vi "configuration UI.vi"() -> ()   [LabVIEW 2013, in "TEC editor node.lvclass"]
uses:
  TEC editor node.lvclass
  <vilib>/NI/Configuration Framework/Node/NodeRef.ctl
  <vilib>/NI/Configuration Framework/Node/NISE_CEF_Node.lvclass
  <vilib>/NI/AMC/Message Queue.ctl
  <vilib>/NI/AMC/Message.ctl
  <vilib>/NI/Tools/Keyed Array/KeyedArray.ctl
  <vilib>/NI/Configuration Framework/Node/UserEventRef.ctl
  <vilib>/NI/Configuration Framework/Controls/EventCluster.ctl
  TEC editor node.lvclass/TEC editor node.ctl
  <vilib>/NI/Tag Bus/tag/Data Type.ctl
  <vilib>/NI/Tag Bus Module Framework/channel/channel classification.ctl
  <vilib>/NI/Tag Bus Module Framework/channel/TBM channel.lvclass/TBM channel.ctl
  <vilib>/NI/Configuration Framework/serializable configuration/NISE_CEF_serializable configuration.lvclass/NISE_CEF_serializable configuration.ctl
  <vilib>/NI/Configuration Framework/serializable configuration/NISE_CEF_serializable configuration.lvclass
  module/configuration/TEC configuration.lvclass
  <vilib>/NI/Tag Bus/tag/tag descriptor.lvclass/tag descriptor.ctl
  <vilib>/NI/Tag Bus Data Framework/Configuration Editor/Classes/Module editor node/Read display name.vi
  <vilib>/NI/Tag Bus Data Framework/Configuration Editor/Classes/Module editor node/module editor node.lvclass
  <vilib>/NI/Configuration Framework/NISE_CEF_TreeControl.lvlib
  <vilib>/NI/Tag Bus/tag/tag descriptor.lvclass
  <vilib>/NI/Module Execution Interface/Engine Configuration/engine configuration.lvclass
  <vilib>/NI/Tag Bus Module Framework/channel/TBM channel.lvclass
  <vilib>/NI/Tag Bus Data Framework/Configuration Editor/Classes/Engine Parent/Engine Parent Editor Node.lvclass
  <vilib>/NI/Tools/Keyed Array/Tools_KeyedArray.lvlib
  <vilib>/NI/AMC/AMC.lvlib
panel:
  in  "Tab Control":enum32{"Module Pairing", "Channel Mapping"}(tab)
  out "Guid":string
  in  "unpair":bool
  out "Paired with":string
  in  "pair":bool
  in  "Pairing Options":i32(listbox)
  in  "remove to":bool
  in  "add to":bool
  in  "toExtList":i32(listbox)
  in  "fromExternallist":i32(listbox)
  in  "avail tags":i32(listbox)=-1
  in  "user event":T1
  in  "main queue":T2
  in  "node ref":T3
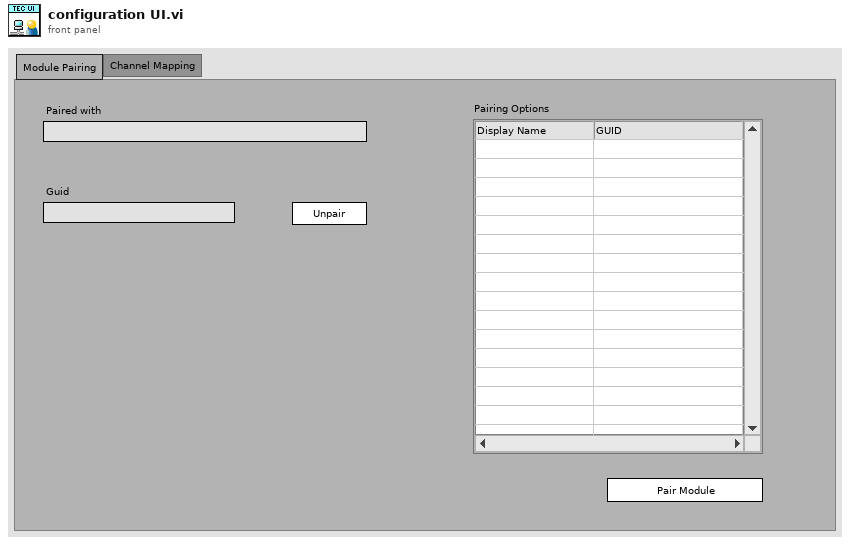
[diagram p1: front panel]
types:
  T1 = typedef "NISE_CEF_Node.lvclass/UserEventRef.ctl" = refnum<user-event>
  T2 = typedef "AMC.lvlib/Message Queue.ctl" = refnum<queue>
  T3 = typedef "NISE_CEF_Node.lvclass/NodeRef.ctl" = refnum<data-value>
  T4 = typedef "NISE_CEF_TreeControl.lvlib/EventCluster.ctl" = cluster{"command":string, "data":string}
  T5 = typedef "TBM channel.lvclass/channel classification.ctl" = enum16{"input data", "output data", "processing parameter", "processing result"}
  T6 = typedef "tag bus.lvlib/tag descriptor.lvclass/Data Type.ctl" = enum16{"Double", "Single", "I64", "I32", "I16", "I8", "U64", "U32", "U16", "U8", "Boolean", "String", "Array of Double", "Array of Single", "Array of I64", "Array of I32", "Array of I16", "Array of I8", "Array of U64", "Array of U32", "Array of U16", "Array of U8", "Array of Boolean", "Array of String"}
  T7 = typedef "TEC editor node.lvclass/pair information.ctl" = cluster{"paired guid":string}
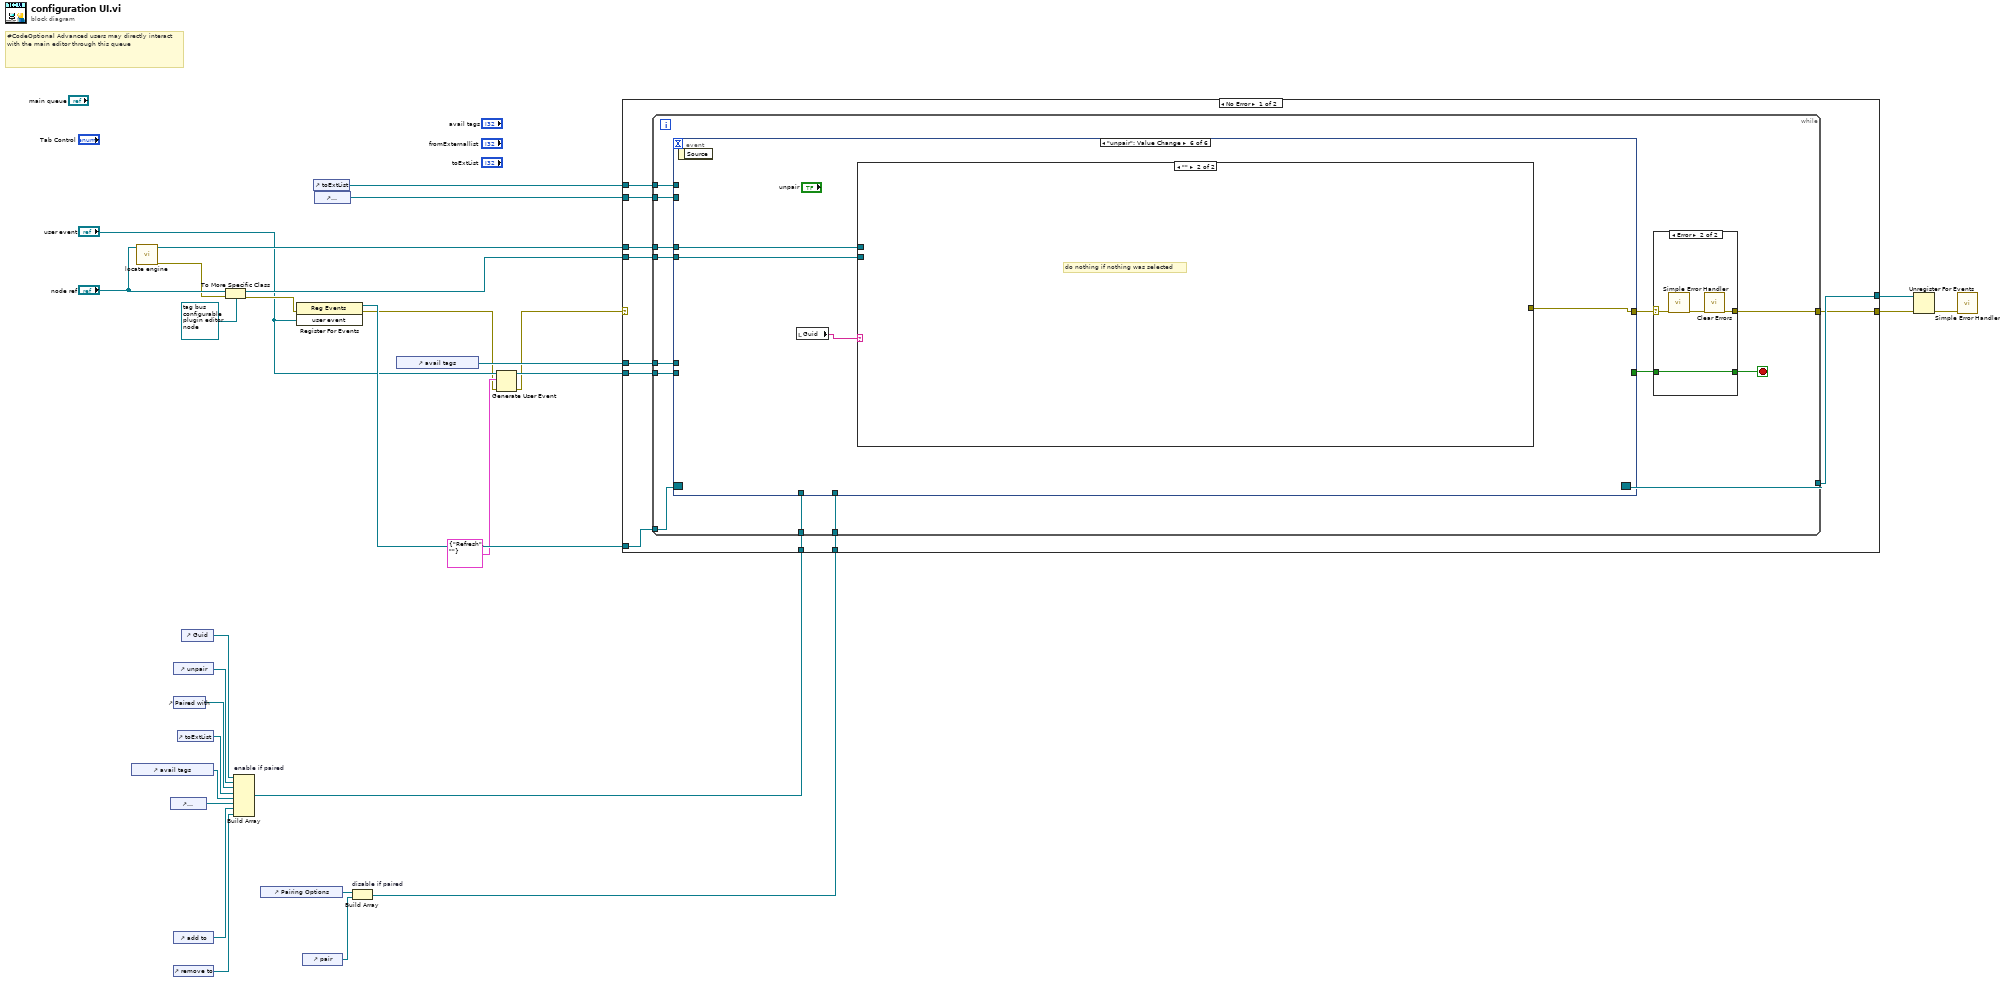
[diagram p0: block diagram]
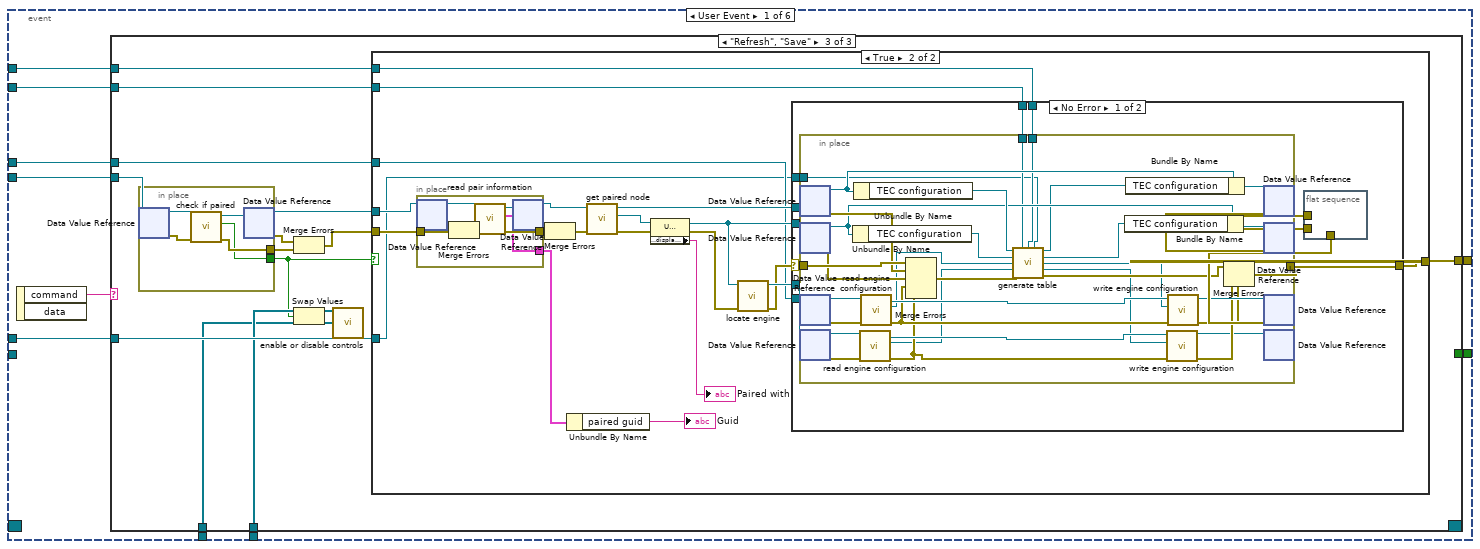
[diagram p3: hidden frame]
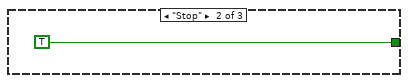
[diagram p5: hidden frame]
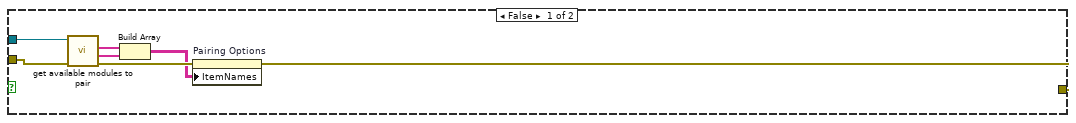
[diagram p6: hidden frame]
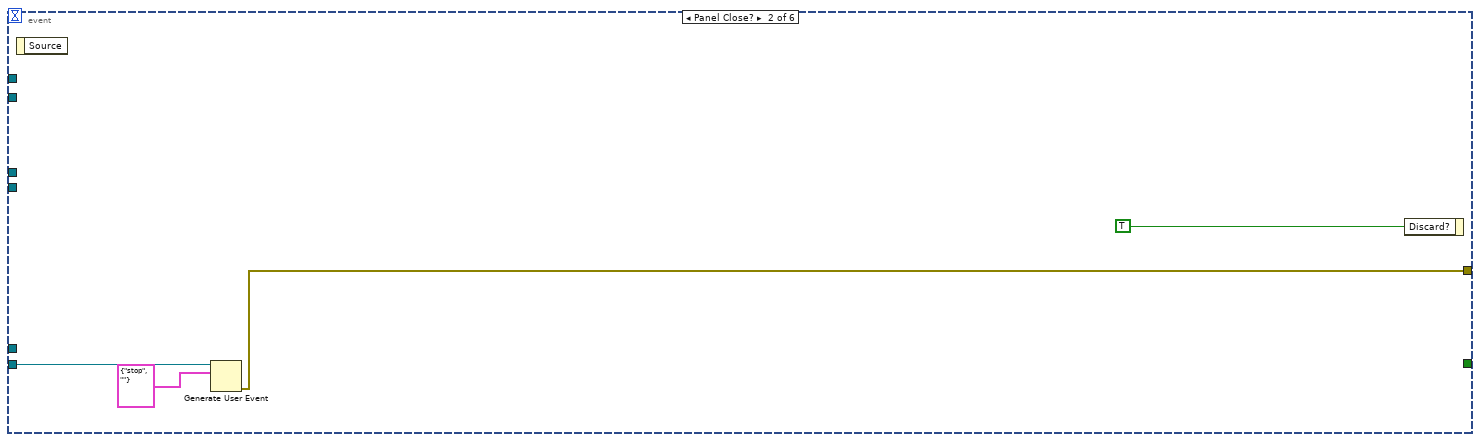
[diagram p8: hidden frame]
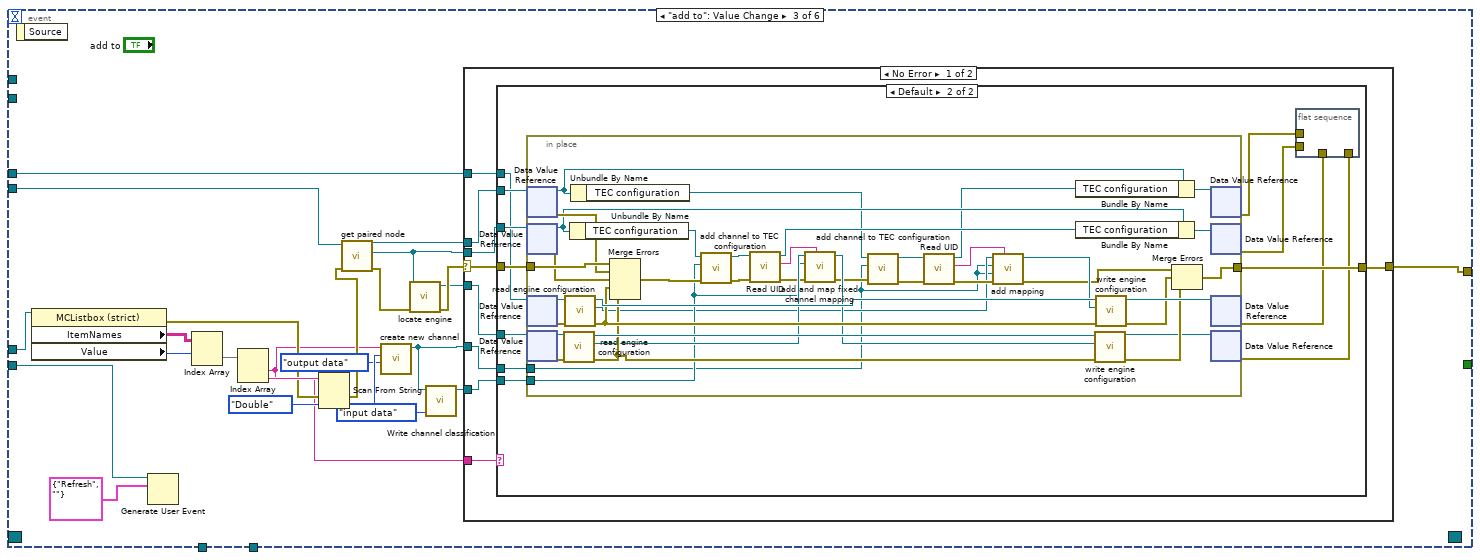
[diagram p9: hidden frame]
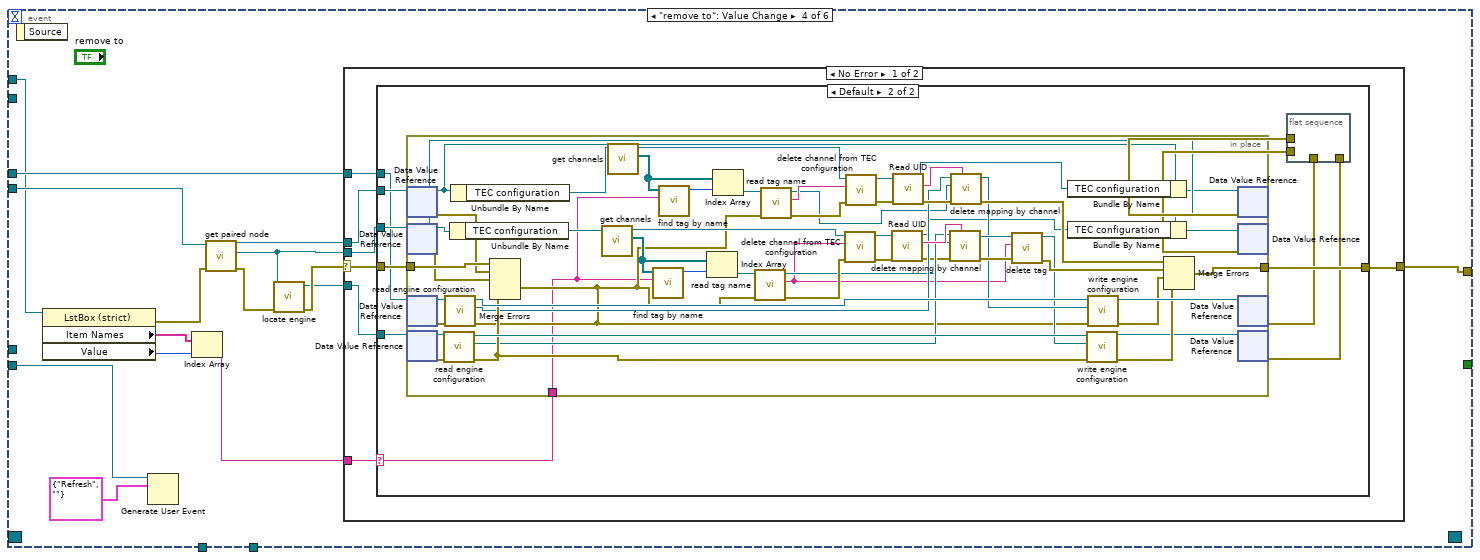
[diagram p12: hidden frame]
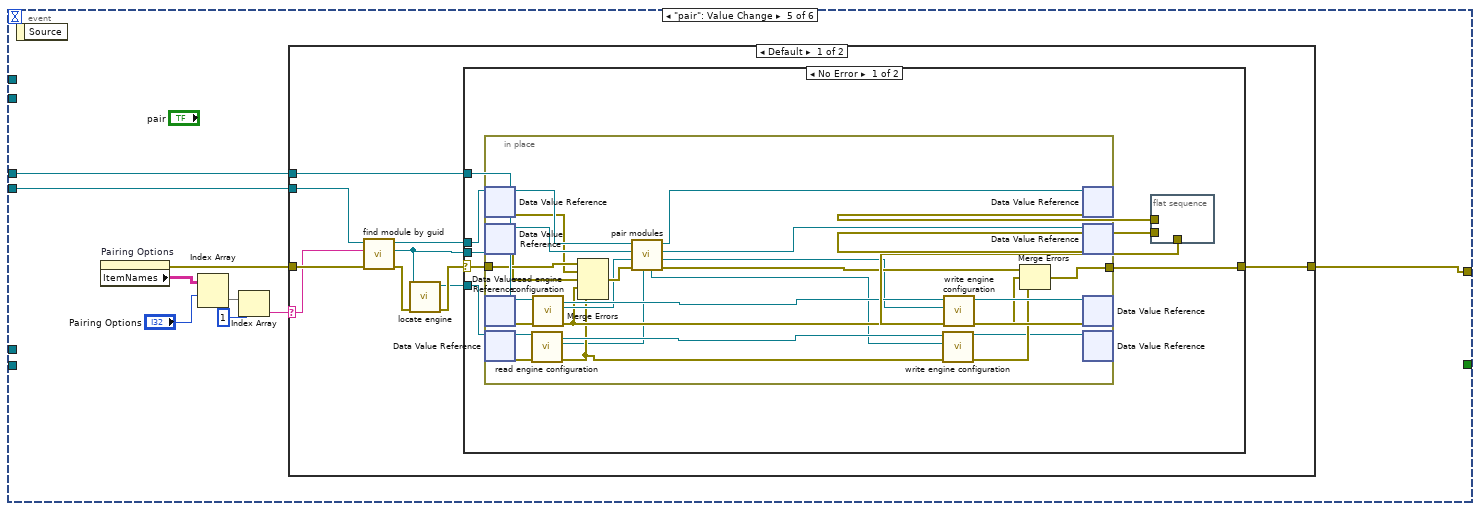
[diagram p15: hidden frame]
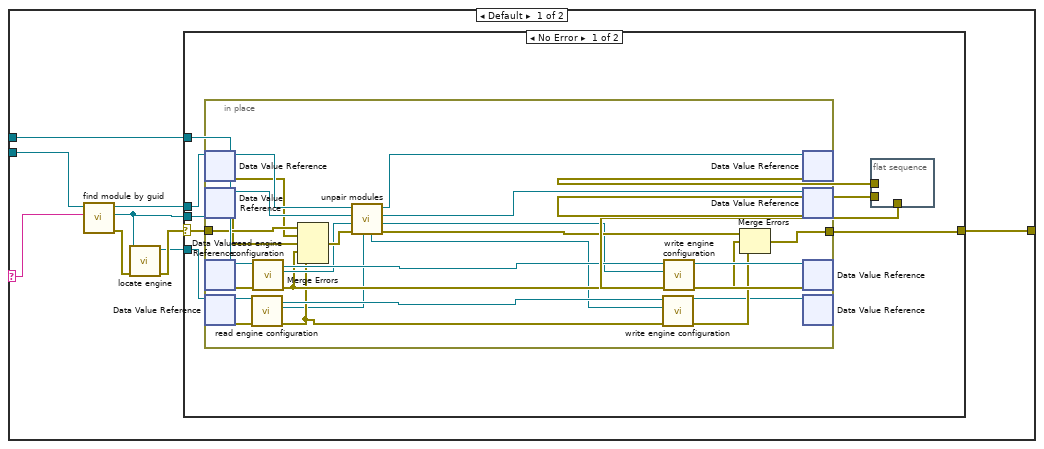
[diagram p18: hidden frame]
diagram:
  # "#CodeOptional Advanced users may directly interact with the main editor through this queue"
  n1 = control-ref of="avail tags"() -> (w10:refnum<vi>)
  n2 = call <vilib>:"locate engine.vi"("component"="node ref") -> ("error out"=w15:errorcluster, "engine"=w23:refnum<data-value>)  [unwired: 9 in]
  n3 = control-ref of="fromExternallist"() -> (w9:refnum<vi>)
  n4 = control-ref of="unpair"() -> (w13:refnum<vi>)
  n5 = control-ref of="Paired with"() -> (w14:refnum<vi>)
  n6 = control-ref of="add to"() -> (w7:refnum<vi>)
  n7 = control-ref of="remove to"() -> (w8:refnum<vi>)
  n8 = control-ref of="toExtList"() -> (w11:refnum<vi>)
  n9 = control-ref of="Guid"() -> (w12:refnum<vi>)
  n10 = To More Specific Class(target class=refnum<data-value> refnum ("data value reference"), reference="node ref", error in=w15) -> (specific class reference=w26:refnum<data-value>, error out=w25:errorcluster)
  n11 = Build Array "enable if paired"(w12, w13, w14, w11, w10, w9, w7, w8) -> (w5:refnum<vi>[])
  n12 = control-ref of="Pairing Options"() -> (w6:refnum<vi>)
  n13 = register-events(error in=w25, "user event") -> (reference out=w30:refnum<event-registration>, error out=w2:errorcluster)  [unwired: 1 in]
  n14 = control-ref of="pair"() -> (w3:refnum<vi>)
  n15 = control-ref of="toExtList"() -> (w21:refnum<vi>)
  n16 = control-ref of="fromExternallist"() -> (w1:refnum<vi>)
  n17 = Build Array "disable if paired"(w6, w3) -> (w4:refnum<vi>[])
  n18 = control-ref of="avail tags"() -> (w22:refnum<vi>)
  n19 = Generate User Event(user event="user event", event data cluster=T4 {"command"="Refresh", "data"=""} ("event data"), error in=w2) -> (user event out=w19:T1, error out=w17:errorcluster)  [unwired: 1 in]
  n20 = case shown="No Error" w17 {
    selector: w17 -> [_ w462]
    tunnel: w30 -> [w41 w461]
    tunnel: [w40 w461] -> w29
    tunnel: [w39 w462] -> w28
    tunnel: w26 -> [w38 _]
    tunnel: w23 -> [w37 _]
    tunnel: w22 -> [w36 _]
    tunnel: w21 -> [w35 _]
    tunnel: w19 -> [w34 _]
    tunnel: w5 -> [w33 _]
    tunnel: w4 -> [w32 _]
    tunnel: w1 -> [w31 _]
    frame No Error {
      n21 = while {
        tunnel: w41 -> [w55]
        tunnel: [w54] -> w40
        tunnel: w38 -> [w49]
        tunnel: w37 -> [w48]
        tunnel: w34 -> [w47]
        tunnel: w36 -> [w46]
        tunnel: w35 -> [w45]
        tunnel: [w50] -> w39
        tunnel: w33 -> [w44]
        tunnel: w32 -> [w43]
        tunnel: w31 -> [w42]
        stop <- w52 stop-if-true
        n22 = event shown="[5] \"unpair\": Value Change" {
          selector: w55 -> [_ _ _ _ _ _]
          dyn-events: [_ _ _ _ _ _] -> w54
          timeout: _ -> [_ _ _ _ _ _]
          tunnel: [w71 _ _ _ _ _] -> w51
          tunnel: [w69 w174 w201 w280 w357 w414] -> w53
          tunnel: w49 -> [w68 _ w197 w276 w359 w415]
          tunnel: w48 -> [w67 _ w200 w279 w356 w413]
          tunnel: w47 -> [_ w175 w192 w271 _ _]
          tunnel: w46 -> [w66 _ w186 _ _ _]
          tunnel: w45 -> [w65 _ _ w268 _ _]
          tunnel: w44 -> [w64 _ _ _ _ _]
          tunnel: w43 -> [w63 _ _ _ _ _]
          tunnel: w42 -> [w62 _ _ _ _ _]
          event User Event {
            n23 = event-data() -> ("command"=w70:string)  [unwired: 1 in, 1 out]
            n24 = case shown="\"Refresh\", \"Save\"" w70 {
              tunnel: [_ TRUE _] -> w71
              tunnel: [_ _ w84] -> w69
              tunnel: w68 -> [_ _ w83]
              tunnel: w67 -> [_ _ w85]
              tunnel: w66 -> [_ _ w87]
              tunnel: w65 -> [_ _ w86]
              tunnel: w64 -> [_ _ w77]
              tunnel: w63 -> [_ _ w78]
              tunnel: w62 -> [_ _ w73]
              frame Default {
              }
              frame "Stop" {
              }
              frame "Refresh", "Save" {
                n25 = in-place {
                  in-place-border: [w170] -> w80
                  in-place-border: [w169] -> w74
                  n26 = in-place-dvr #1(w83) -> (w173:refnum<class "TEC editor node.lvclass">, w171:errorcluster)
                  n27 = call "check if paired.vi"("error in"=w171, "UDP Broadcast Editor Node in"=w173) -> ("error out"=w170:errorcluster, "paired"=w169:bool, "UDP Broadcast Editor Node out"=w172:refnum<class "TEC editor node.lvclass">)  [unwired: 7 in]
                  n28 = in-place-dvr #1(w172) -> (w82:refnum<data-value>, w81:errorcluster)
                }
                n29 = Merge Errors(w81, w80) -> (w75:errorcluster)
                n30 = Swap Values(12:w78, 13:w74, 14:w77) -> (1:w79:refnum<vi>[], 3:w76:refnum<vi>[])
                n31 = call "enable or disable controls.vi"("disable set"=w76, "enable set"=w79) -> ()  [unwired: 10 in]
                n32 = case shown="True" w74 {
                  tunnel: w87 -> [_ w95]
                  tunnel: w86 -> [_ w96]
                  tunnel: w85 -> [_ w98]
                  tunnel: [w88 w102] -> w84
                  tunnel: w82 -> [w94 w105]
                  tunnel: w75 -> [w93 w106]
                  tunnel: w73 -> [_ w97]
                  frame False {
                    n33 = call "get available modules to pair.vi"("error in"=w93, "editor in"=w94) -> ("error out"=w90:errorcluster, "Display Name"=w92:string[], "IDs"=w91:string[])  [unwired: 6 in, 1 out]
                    n34 = Build Array(w91, w92) -> (w89:string[][])
                    n35 = property on="Pairing Options" class="MCListbox (strict)"(error in=w90, "ItemNames"=w89) -> (error out=w88:errorcluster)  [unwired: 1 in, 1 out]
                  }
                  frame True {
                    n36 = in-place {
                      in-place-border: w106 -> [w164]
                      in-place-border: [w168] -> w113
                      in-place-border: [w162] -> w108
                      n37 = in-place-dvr #2(w105) -> (w167:refnum<class "TEC editor node.lvclass">, w163:errorcluster)
                      n38 = Merge Errors(w164, w163) -> (w165:errorcluster)
                      n39 = call "read pair information.vi"("error in"=w165, "UDP Broadcast Editor Node in"=w167) -> ("error out"=w168:errorcluster, "pair info"=w162:T7, "UDP Broadcast Editor Node out"=w166:refnum<class "TEC editor node.lvclass">)  [unwired: 7 in]
                      n40 = in-place-dvr #2(w166) -> (w115:refnum<data-value>, w112:errorcluster)
                    }
                    n41 = Merge Errors(w113, w112) -> (w114:errorcluster)
                    n42 = Unbundle By Name(w108) -> ("paired guid"=→"Guid":string)
                    n43 = call "get paired node.vi"("error in"=w114, "editor in"=w115) -> ("error out"=w110:errorcluster, "paired node"=w111:refnum<data-value>, "editor out"=w100:refnum<data-value>)  [unwired: 7 in]
                    n44 = property class="UDP Broadcast Editor Node"(reference=w111, error in=w110) -> (reference out=w99:refnum<data-value>, error out=w101:errorcluster, "Data Access:display name"=→"Paired with":string)
                    n45 = call <vilib>:"locate engine.vi"("error in"=w101, "component"=w99) -> ("error out"=w103:errorcluster, "engine"=w104:refnum<data-value>)  [unwired: 8 in]
                    n46 = case shown="No Error" w103 {
                      selector: w103 -> [w127 w161]
                      tunnel: [w126 w161] -> w102
                      tunnel: w104 -> [w122 _]
                      tunnel: w100 -> [w121 _]
                      tunnel: w99 -> [w120 _]
                      tunnel: w98 -> [w119 _]
                      tunnel: w97 -> [w118 _]
                      tunnel: w96 -> [w117 _]
                      tunnel: w95 -> [w116 _]
                      frame No Error {
                        n47 = in-place {
                          in-place-border: w127 -> [w160]
                          in-place-border: [w153] -> w126
                          in-place-border: w118 -> [w130]
                          in-place-border: w117 -> [w129]
                          in-place-border: w116 -> [w128]
                          n48 = in-place-dvr #3(w121) -> (w136:refnum<class "TEC editor node.lvclass">, w159:errorcluster)
                          n49 = in-place-dvr #4(w120) -> (w133:refnum<class "TEC editor node.lvclass">, w158:errorcluster)
                          n50 = in-place-dvr #5(w119) -> (w157:refnum<class "Engine Parent Editor Node.lvclass">, w156:errorcluster)
                          n51 = in-place-dvr #6(w122) -> (w149:refnum<class "Engine Parent Editor Node.lvclass">, w148:errorcluster)
                          n52 = Unbundle By Name(w133) -> ("TEC configuration"=w137:refnum<class "TEC configuration.lvclass">)
                          n53 = Unbundle By Name(w136) -> ("TEC configuration"=w138:refnum<class "TEC configuration.lvclass">)
                          n54 = call <vilib>:"read engine configuration.vi"("error in"=w148, "Engine Parent Editor Node in"=w149) -> ("error out"=w147:errorcluster, "engine configuration"=w140:refnum<class "engine configuration.lvclass">, "Engine Parent Editor Node out"=w150:refnum<class "Engine Parent Editor Node.lvclass">)  [unwired: 7 in]
                          n55 = call <vilib>:"read engine configuration.vi"("error in"=w156, "Engine Parent Editor Node in"=w157) -> ("error out"=w151:errorcluster, "engine configuration"=w139:refnum<class "engine configuration.lvclass">, "Engine Parent Editor Node out"=w155:refnum<class "Engine Parent Editor Node.lvclass">)  [unwired: 7 in]
                          n56 = Merge Errors(w160, w159, w158, w151, w147) -> (w144:errorcluster)
                          n57 = call "generate table.vi"("TEC in"=w138, "from TEC"=w130, "to TEC"=w129, "avail tags"=w128, "Pair in"=w137, "engine configuration in"=w139, "paired engine in"=w140, "error in"=w144) -> ("TEC out"=w131:refnum<class "TEC configuration.lvclass">, "pair out"=w132:refnum<class "TEC configuration.lvclass">, "engine configuration out"=w141:refnum<class "engine configuration.lvclass">, "paired engine out"=w142:refnum<class "engine configuration.lvclass">, "error out"=w143:errorcluster)  [unwired: 3 in]
                          n58 = Bundle By Name(cluster=w133, "TEC configuration"=w132) -> (w134:refnum<class "TEC editor node.lvclass">)
                          n59 = Bundle By Name(cluster=w136, "TEC configuration"=w131) -> (w135:refnum<class "TEC editor node.lvclass">)
                          n60 = call <vilib>:"write engine configuration.vi"("error in"=w147, "engine configuration"=w142, "Engine Parent Editor Node in"=w150) -> ("error out"=w146:errorcluster, "Engine Parent Editor Node out"=w145:refnum<class "Engine Parent Editor Node.lvclass">)  [unwired: 7 in]
                          n61 = call <vilib>:"write engine configuration.vi"("error in"=w151, "engine configuration"=w141, "Engine Parent Editor Node in"=w155) -> ("error out"=w152:errorcluster, "Engine Parent Editor Node out"=w154:refnum<class "Engine Parent Editor Node.lvclass">)  [unwired: 7 in]
                          n62 = Merge Errors(w143, w152, w146) -> (w153:errorcluster)
                          n63 = in-place-dvr #3(w135) -> (w125:errorcluster)  [unwired: 1 out]
                          n64 = in-place-dvr #4(w134) -> (w124:errorcluster)  [unwired: 1 out]
                          n65 = in-place-dvr #5(w154) -> (w123:errorcluster)  [unwired: 1 out]
                          n66 = in-place-dvr #6(w145) -> ()  [unwired: 2 out]
                        }
                        n67 = flat-sequence {
                          tunnel: w125 -> [_]
                          tunnel: w124 -> [_]
                          tunnel: w123 -> [_]
                          frame #0 {
                          }
                        }
                      }
                      frame Error {
                      }
                    }
                  }
                }
              }
            }
          }
          event Panel Close? {
            n68 = event-data() -> ()  [unwired: 1 in, 1 out]
            n69 = Generate User Event(user event=w175, event data cluster=T4 {"command"="stop", "data"=""} ("event data")) -> (error out=w174:errorcluster)  [unwired: 2 in, 1 out]
            n70 = event-data("Discard?"=TRUE) -> ()  [unwired: 1 in, 1 out]
          }
          event "add to": Value Change {
            n71 = event-data() -> ()  [unwired: 1 in, 1 out]
            n72 = property class="MCListbox (strict)"(reference=w186) -> (error out=w184:errorcluster, "ItemNames"=w191:string[][], "Value"=w190:i32)  [unwired: 1 in, 1 out]
            n73 = Generate User Event(user event=w192, event data cluster=T4 {"command"="Refresh", "data"=""} ("event data")) -> ()  [unwired: 2 in, 2 out]
            n74 = Index Array(array=w191, index (row)=w190) -> (element=w187:string[])  [unwired: 1 in]
            n75 = Index Array(array=w187) -> (element #1=w178:string, element #2=w189:string)  [unwired: 2 in]
            n76 = Scan From String(input string=w189, error in=w184, default 1=Data_Type."Double" ("data type")) -> (error out=w185:errorcluster, output 1=w183:T6)  [unwired: 2 in, 2 out]
            n77 = call "get paired node.vi"("error in"=w185, "editor in"=w197) -> ("error out"=w194:errorcluster, "paired node"=w195:refnum<data-value>, "editor out"=w196:refnum<data-value>)  [unwired: 7 in]
            n78 = call <vilib>:"create new channel.vi"("channel classification"=channel_classification."output data", "data type"=w183, "channel name"=w178) -> ("channel"=w181:refnum<class "TBM channel.lvclass">)  [unwired: 8 in]
            n79 = call <vilib>:"locate engine.vi"("error in"=w194, "component"=w195) -> ("error out"=w199:errorcluster, "engine"=w198:refnum<data-value>)  [unwired: 8 in]
            n80 = call <vilib>:"Write channel classification.vi"("channel classification"=channel_classification."input data", "channel in"=w181) -> ("channel out"=w180:refnum<class "TBM channel.lvclass">)  [unwired: 8 in, 1 out]
            n81 = case shown="No Error" w199 {
              selector: w199 -> [w210 w265]
              tunnel: [w209 w265] -> w201
              tunnel: w196 -> [w208 _]
              tunnel: w195 -> [w207 _]
              tunnel: w200 -> [w206 _]
              tunnel: w198 -> [w205 _]
              tunnel: w181 -> [w202 _]
              tunnel: w180 -> [w203 _]
              tunnel: w178 -> [w204 _]
              frame No Error {
                n82 = case shown="Default" w204 {
                  tunnel: w210 -> [w211 w223]
                  tunnel: [w211 w222] -> w209
                  tunnel: w208 -> [_ w221]
                  tunnel: w207 -> [_ w220]
                  tunnel: w206 -> [_ w219]
                  tunnel: w205 -> [_ w216]
                  tunnel: w203 -> [_ w213]
                  tunnel: w202 -> [_ w212]
                  frame "" {
                  }
                  frame Default {
                    n83 = in-place {
                      in-place-border: w223 -> [w264]
                      in-place-border: [w257] -> w222
                      in-place-border: w213 -> [w242]
                      in-place-border: w212 -> [w226]
                      n84 = in-place-dvr #7(w221) -> (w247:refnum<class "TEC editor node.lvclass">, w263:errorcluster)
                      n85 = in-place-dvr #8(w220) -> (w246:refnum<class "TEC editor node.lvclass">, w262:errorcluster)
                      n86 = in-place-dvr #9(w219) -> (w261:refnum<class "Engine Parent Editor Node.lvclass">, w260:errorcluster)
                      n87 = in-place-dvr #10(w216) -> (w253:refnum<class "Engine Parent Editor Node.lvclass">, w252:errorcluster)
                      n88 = call <vilib>:"read engine configuration.vi"("error in"=w252, "Engine Parent Editor Node in"=w253) -> ("error out"=w251:errorcluster, "engine configuration"=w243:refnum<class "engine configuration.lvclass">, "Engine Parent Editor Node out"=w254:refnum<class "Engine Parent Editor Node.lvclass">)  [unwired: 7 in]
                      n89 = call <vilib>:"read engine configuration.vi"("error in"=w260, "Engine Parent Editor Node in"=w261) -> ("error out"=w255:errorcluster, "engine configuration"=w228:refnum<class "engine configuration.lvclass">, "Engine Parent Editor Node out"=w259:refnum<class "Engine Parent Editor Node.lvclass">)  [unwired: 7 in]
                      n90 = Unbundle By Name(w246) -> ("TEC configuration"=w244:refnum<class "TEC configuration.lvclass">)
                      n91 = Unbundle By Name(w247) -> ("TEC configuration"=w234:refnum<class "TEC configuration.lvclass">)
                      n92 = Merge Errors(w264, w263, w262, w255, w251) -> (w248:errorcluster)
                      n93 = call "add channel to TEC configuration.vi"("error in"=w248, "channel"=w242, "TEC configuration in"=w244) -> ("error out"=w241:errorcluster, "TEC configuration out"=w240:refnum<class "TEC configuration.lvclass">)  [unwired: 7 in]
                      n94 = call <vilib>:"Read UID.vi"("error in"=w241, "configuration in"=w240) -> ("error out"=w239:errorcluster, "instance id"=w238:string, "configuration out"=w237:refnum<class "TEC configuration.lvclass">)  [unwired: 7 in]
                      n95 = call <vilib>:"add and map fixed channel mapping.vi"("module instance"=w238, "error in"=w239, "fixed channel"=w242, "engine configuration in"=w243) -> ("error out"=w235:errorcluster, "engine configuration out"=w236:refnum<class "engine configuration.lvclass">)  [unwired: 6 in]
                      n96 = call "add channel to TEC configuration.vi"("error in"=w235, "channel"=w226, "TEC configuration in"=w234) -> ("error out"=w232:errorcluster, "TEC configuration out"=w233:refnum<class "TEC configuration.lvclass">)  [unwired: 7 in]
                      n97 = call <vilib>:"Read UID.vi"("error in"=w232, "configuration in"=w233) -> ("error out"=w231:errorcluster, "instance id"=w227:string, "configuration out"=w230:refnum<class "TEC configuration.lvclass">)  [unwired: 7 in]
                      n98 = call <vilib>:"add mapping.vi"("owner ID"=w227, "error in"=w231, "channel"=w226, "tag descriptor"=w226, "engine configuration"=w228) -> ("error out"=w225:errorcluster, "engine configuration out"=w229:refnum<class "engine configuration.lvclass">)  [unwired: 5 in]
                      n99 = Bundle By Name(cluster=w247, "TEC configuration"=w230) -> (w224:refnum<class "TEC editor node.lvclass">)
                      n100 = Bundle By Name(cluster=w246, "TEC configuration"=w237) -> (w245:refnum<class "TEC editor node.lvclass">)
                      n101 = call <vilib>:"write engine configuration.vi"("error in"=w251, "engine configuration"=w236, "Engine Parent Editor Node in"=w254) -> ("error out"=w250:errorcluster, "Engine Parent Editor Node out"=w249:refnum<class "Engine Parent Editor Node.lvclass">)  [unwired: 7 in]
                      n102 = call <vilib>:"write engine configuration.vi"("error in"=w255, "engine configuration"=w229, "Engine Parent Editor Node in"=w259) -> ("error out"=w256:errorcluster, "Engine Parent Editor Node out"=w258:refnum<class "Engine Parent Editor Node.lvclass">)  [unwired: 7 in]
                      n103 = Merge Errors(w225, w256, w250) -> (w257:errorcluster)
                      n104 = in-place-dvr #7(w224) -> (w218:errorcluster)  [unwired: 1 out]
                      n105 = in-place-dvr #8(w245) -> (w217:errorcluster)  [unwired: 1 out]
                      n106 = in-place-dvr #9(w258) -> (w215:errorcluster)  [unwired: 1 out]
                      n107 = in-place-dvr #10(w249) -> (w214:errorcluster)  [unwired: 1 out]
                    }
                    n108 = flat-sequence {
                      tunnel: w218 -> [_]
                      tunnel: w217 -> [_]
                      tunnel: w215 -> [_]
                      tunnel: w214 -> [_]
                      frame #0 {
                      }
                    }
                  }
                }
              }
              frame Error {
              }
            }
          }
          event "remove to": Value Change {
            n109 = event-data() -> ()  [unwired: 1 in, 1 out]
            n110 = property class="LstBox (strict)"(reference=w268) -> (error out=w267:errorcluster, "Item Names"=w270:string[], "Value"=w269:i32)  [unwired: 1 in, 1 out]
            n111 = Generate User Event(user event=w271, event data cluster=T4 {"command"="Refresh", "data"=""} ("event data")) -> ()  [unwired: 2 in, 2 out]
            n112 = Index Array(array=w270, index=w269) -> (element=w266:string)
            n113 = call "get paired node.vi"("error in"=w267, "editor in"=w276) -> ("error out"=w273:errorcluster, "paired node"=w274:refnum<data-value>, "editor out"=w275:refnum<data-value>)  [unwired: 7 in]
            n114 = call <vilib>:"locate engine.vi"("error in"=w273, "component"=w274) -> ("error out"=w278:errorcluster, "engine"=w277:refnum<data-value>)  [unwired: 8 in]
            n115 = case shown="No Error" w278 {
              selector: w278 -> [w287 w355]
              tunnel: [w286 w355] -> w280
              tunnel: w275 -> [w285 _]
              tunnel: w274 -> [w284 _]
              tunnel: w279 -> [w283 _]
              tunnel: w277 -> [w282 _]
              tunnel: w266 -> [w281 _]
              frame No Error {
                n116 = case shown="Default" w281 {
                  selector: w281 -> [_ w289]
                  tunnel: w287 -> [w288 w299]
                  tunnel: [w288 w298] -> w286
                  tunnel: w285 -> [_ w297]
                  tunnel: w284 -> [_ w296]
                  tunnel: w283 -> [_ w295]
                  tunnel: w282 -> [_ w292]
                  frame "" {
                  }
                  frame Default {
                    n117 = in-place {
                      in-place-border: w299 -> [w354]
                      in-place-border: [w347] -> w298
                      in-place-border: w289 -> [w301]
                      n118 = in-place-dvr #11(w297) -> (w339:refnum<class "TEC editor node.lvclass">, w353:errorcluster)
                      n119 = in-place-dvr #12(w296) -> (w338:refnum<class "TEC editor node.lvclass">, w352:errorcluster)
                      n120 = in-place-dvr #13(w295) -> (w351:refnum<class "Engine Parent Editor Node.lvclass">, w350:errorcluster)
                      n121 = in-place-dvr #14(w292) -> (w344:refnum<class "Engine Parent Editor Node.lvclass">, w343:errorcluster)
                      n122 = call <vilib>:"read engine configuration.vi"("error in"=w343, "Engine Parent Editor Node in"=w344) -> ("error out"=w342:errorcluster, "engine configuration"=w324:refnum<class "engine configuration.lvclass">, "Engine Parent Editor Node out"=w345:refnum<class "Engine Parent Editor Node.lvclass">)  [unwired: 7 in]
                      n123 = call <vilib>:"read engine configuration.vi"("error in"=w350, "Engine Parent Editor Node in"=w351) -> ("error out"=w307:errorcluster, "engine configuration"=w323:refnum<class "engine configuration.lvclass">, "Engine Parent Editor Node out"=w349:refnum<class "Engine Parent Editor Node.lvclass">)  [unwired: 7 in]
                      n124 = Unbundle By Name(w338) -> ("TEC configuration"=w314:refnum<class "TEC configuration.lvclass">)
                      n125 = Unbundle By Name(w339) -> ("TEC configuration"=w312:refnum<class "TEC configuration.lvclass">)
                      n126 = Merge Errors(w354, w353, w352, w307, w342) -> ()  [unwired: 1 out]
                      n127 = call-dynamic "get channels.vi"("TEC configuration in"=w314) -> ("channels"=w316:refnum<class "TBM channel.lvclass">[], "TEC configuration out"=w313:refnum<class "TEC configuration.lvclass">)  [unwired: 9 in]
                      n128 = call-dynamic "get channels.vi"("TEC configuration in"=w312) -> ("channels"=w319:refnum<class "TBM channel.lvclass">[], "TEC configuration out"=w311:refnum<class "TEC configuration.lvclass">)  [unwired: 9 in]
                      n129 = call <vilib>:"find tag by name.vi"("name"=w301, "tags in"=w316) -> ("index"=w315:i32)  [unwired: 9 in]
                      n130 = call <vilib>:"find tag by name.vi"("name"=w301, "tags in"=w319) -> ("index"=w318:i32)  [unwired: 9 in]
                      n131 = Index Array(array=w316, index=w315) -> (element=w317:refnum<class "TBM channel.lvclass">)
                      n132 = Index Array(array=w319, index=w318) -> (element=w320:refnum<class "TBM channel.lvclass">)
                      n133 = call <vilib>:"read tag name.vi"("error in"=w307, "system tag in"=w317) -> ("error out"=w308:errorcluster, "name"=w302:string, "system tag out"=w304:refnum<class "TBM channel.lvclass">)  [unwired: 7 in]
                      n134 = call <vilib>:"read tag name.vi"("error in"=w307, "system tag in"=w320) -> ("error out"=w309:errorcluster, "name"=w310:string, "system tag out"=w305:refnum<class "TBM channel.lvclass">)  [unwired: 7 in]
                      n135 = call "delete channel from TEC configuration.vi"("error in"=w308, "channel to delete"=w302, "TEC configuration in"=w313) -> ("error out"=w306:errorcluster, "TEC configuration out"=w333:refnum<class "TEC configuration.lvclass">)  [unwired: 7 in]
                      n136 = call "delete channel from TEC configuration.vi"("error in"=w309, "channel to delete"=w310, "TEC configuration in"=w311) -> ("error out"=w335:errorcluster, "TEC configuration out"=w336:refnum<class "TEC configuration.lvclass">)  [unwired: 7 in]
                      n137 = call <vilib>:"Read UID.vi"("error in"=w306, "configuration in"=w333) -> ("error out"=w303:errorcluster, "instance id"=w330:string, "configuration out"=w321:refnum<class "TEC configuration.lvclass">)  [unwired: 7 in]
                      n138 = call <vilib>:"Read UID.vi"("error in"=w335, "configuration in"=w336) -> ("error out"=w334:errorcluster, "instance id"=w329:string, "configuration out"=w322:refnum<class "TEC configuration.lvclass">)  [unwired: 7 in]
                      n139 = call <vilib>:"delete mapping by channel.vi"("owner ID"=w330, "error in"=w303, "channel"=w304, "engine configuration in"=w324) -> ("error out"=w331:errorcluster, "engine configuration out"=w332:refnum<class "engine configuration.lvclass">)  [unwired: 6 in]
                      n140 = call <vilib>:"delete mapping by channel.vi"("owner ID"=w329, "error in"=w334, "channel"=w305, "engine configuration in"=w323) -> ("error out"=w327:errorcluster, "engine configuration out"=w326:refnum<class "engine configuration.lvclass">)  [unwired: 6 in]
                      n141 = call <vilib>:"delete tag.vi"("error in"=w331, "tag name"=w302, "engine configuration in"=w332) -> ("error out"=w328:errorcluster, "engine configuration out"=w325:refnum<class "engine configuration.lvclass">)  [unwired: 7 in]
                      n142 = Bundle By Name(cluster=w339, "TEC configuration"=w322) -> (w300:refnum<class "TEC editor node.lvclass">)
                      n143 = Bundle By Name(cluster=w338, "TEC configuration"=w321) -> (w337:refnum<class "TEC editor node.lvclass">)
                      n144 = call <vilib>:"write engine configuration.vi"("error in"=w342, "engine configuration"=w325, "Engine Parent Editor Node in"=w345) -> ("error out"=w341:errorcluster, "Engine Parent Editor Node out"=w340:refnum<class "Engine Parent Editor Node.lvclass">)  [unwired: 7 in]
                      n145 = call <vilib>:"write engine configuration.vi"("error in"=w307, "engine configuration"=w326, "Engine Parent Editor Node in"=w349) -> ("error out"=w346:errorcluster, "Engine Parent Editor Node out"=w348:refnum<class "Engine Parent Editor Node.lvclass">)  [unwired: 7 in]
                      n146 = Merge Errors(w327, w328, w346, w341) -> (w347:errorcluster)
                      n147 = in-place-dvr #11(w300) -> (w294:errorcluster)  [unwired: 1 out]
                      n148 = in-place-dvr #12(w337) -> (w293:errorcluster)  [unwired: 1 out]
                      n149 = in-place-dvr #13(w348) -> (w291:errorcluster)  [unwired: 1 out]
                      n150 = in-place-dvr #14(w340) -> (w290:errorcluster)  [unwired: 1 out]
                    }
                    n151 = flat-sequence {
                      tunnel: w294 -> [_]
                      tunnel: w293 -> [_]
                      tunnel: w291 -> [_]
                      tunnel: w290 -> [_]
                      frame #0 {
                      }
                    }
                  }
                }
              }
              frame Error {
              }
            }
          }
          event "pair": Value Change {
            n152 = event-data() -> ()  [unwired: 1 in, 1 out]
            n153 = property on="Pairing Options" class="MCListbox (strict)"() -> (error out=w358:errorcluster, "ItemNames"=w364:string[][])  [unwired: 2 in, 1 out]
            n154 = Index Array(array=w364, index (row)="Pairing Options") -> (element=w362:string[])  [unwired: 1 in]
            n155 = Index Array(array=w362, index=1) -> (element=w360:string)
            n156 = case shown="Default" w360 {
              selector: w360 -> [w372 _]
              tunnel: w359 -> [w374 _]
              tunnel: w358 -> [w373 w411]
              tunnel: [w371 w411] -> w357
              tunnel: w356 -> [w369 _]
              frame Default {
                n157 = call "find module by guid.vi"("error in (no error)"=w373, "GUID"=w372, "ME in"=w374) -> ("error out"=w368:errorcluster, "UDP refs"=w366:refnum<data-value>, "ME out"=w370:refnum<data-value>)  [unwired: 6 in]
                n158 = call <vilib>:"locate engine.vi"("error in"=w368, "component"=w366) -> ("error out"=w367:errorcluster, "engine"=w365:refnum<data-value>)  [unwired: 8 in]
                n159 = case shown="No Error" w367 {
                  selector: w367 -> [w383 w410]
                  tunnel: [w382 w410] -> w371
                  tunnel: w370 -> [w381 _]
                  tunnel: w366 -> [w380 _]
                  tunnel: w369 -> [w379 _]
                  tunnel: w365 -> [w375 _]
                  frame No Error {
                    n160 = in-place {
                      in-place-border: w383 -> [w409]
                      in-place-border: [w394] -> w382
                      n161 = in-place-dvr #15(w381) -> (w406:refnum<class "TEC editor node.lvclass">, w404:errorcluster)
                      n162 = in-place-dvr #16(w380) -> (w407:refnum<class "TEC editor node.lvclass">, w403:errorcluster)
                      n163 = in-place-dvr #17(w379) -> (w400:refnum<class "Engine Parent Editor Node.lvclass">, w399:errorcluster)
                      n164 = in-place-dvr #18(w375) -> (w390:refnum<class "Engine Parent Editor Node.lvclass">, w389:errorcluster)
                      n165 = call <vilib>:"read engine configuration.vi"("error in"=w389, "Engine Parent Editor Node in"=w390) -> ("error out"=w388:errorcluster, "engine configuration"=w384:refnum<class "engine configuration.lvclass">, "Engine Parent Editor Node out"=w391:refnum<class "Engine Parent Editor Node.lvclass">)  [unwired: 7 in]
                      n166 = call <vilib>:"read engine configuration.vi"("error in"=w399, "Engine Parent Editor Node in"=w400) -> ("error out"=w392:errorcluster, "engine configuration"=w396:refnum<class "engine configuration.lvclass">, "Engine Parent Editor Node out"=w398:refnum<class "Engine Parent Editor Node.lvclass">)  [unwired: 7 in]
                      n167 = Merge Errors(w409, w404, w403, w392, w388) -> (w405:errorcluster)
                      n168 = call "pair modules.vi"("paired engine in"=w384, "error in"=w405, "engine configuration in"=w396, "module to pair with"=w407, "UDP Broadcast Editor Node in"=w406) -> ("error out"=w408:errorcluster, "engine configuration out"=w395:refnum<class "engine configuration.lvclass">, "module to pair with out"=w401:refnum<class "TEC editor node.lvclass">, "UDP Broadcast Editor Node out"=w402:refnum<class "TEC editor node.lvclass">, "paired engine out"=w385:refnum<class "engine configuration.lvclass">)  [unwired: 2 in]
                      n169 = call <vilib>:"write engine configuration.vi"("error in"=w388, "engine configuration"=w385, "Engine Parent Editor Node in"=w391) -> ("error out"=w387:errorcluster, "Engine Parent Editor Node out"=w386:refnum<class "Engine Parent Editor Node.lvclass">)  [unwired: 7 in]
                      n170 = call <vilib>:"write engine configuration.vi"("error in"=w392, "engine configuration"=w395, "Engine Parent Editor Node in"=w398) -> ("error out"=w393:errorcluster, "Engine Parent Editor Node out"=w397:refnum<class "Engine Parent Editor Node.lvclass">)  [unwired: 7 in]
                      n171 = Merge Errors(w408, w393, w387) -> (w394:errorcluster)
                      n172 = in-place-dvr #15(w402) -> (w378:errorcluster)  [unwired: 1 out]
                      n173 = in-place-dvr #16(w401) -> (w377:errorcluster)  [unwired: 1 out]
                      n174 = in-place-dvr #17(w397) -> (w376:errorcluster)  [unwired: 1 out]
                      n175 = in-place-dvr #18(w386) -> ()  [unwired: 2 out]
                    }
                    n176 = flat-sequence {
                      tunnel: w378 -> [_]
                      tunnel: w377 -> [_]
                      tunnel: w376 -> [_]
                      frame #0 {
                      }
                    }
                  }
                  frame Error {
                  }
                }
              }
              frame "" {
                # "do nothing if nothing was selected"
              }
            }
          }
          event "unpair": Value Change {
            n177 = event-data() -> ()  [unwired: 1 in, 1 out]
            n178 = local read "Guid"() -> (w412:string)
            n179 = case shown="\"\"" w412 {
              selector: w412 -> [w423 _]
              tunnel: w415 -> [w424 _]
              tunnel: [w422 _] -> w414
              tunnel: w413 -> [w420 _]
              frame Default {
                n180 = call "find module by guid.vi"("GUID"=w423, "ME in"=w424) -> ("error out"=w419:errorcluster, "UDP refs"=w417:refnum<data-value>, "ME out"=w421:refnum<data-value>)  [unwired: 7 in]
                n181 = call <vilib>:"locate engine.vi"("error in"=w419, "component"=w417) -> ("error out"=w418:errorcluster, "engine"=w416:refnum<data-value>)  [unwired: 8 in]
                n182 = case shown="No Error" w418 {
                  selector: w418 -> [w433 w460]
                  tunnel: [w432 w460] -> w422
                  tunnel: w421 -> [w431 _]
                  tunnel: w417 -> [w430 _]
                  tunnel: w420 -> [w429 _]
                  tunnel: w416 -> [w425 _]
                  frame No Error {
                    n183 = in-place {
                      in-place-border: w433 -> [w459]
                      in-place-border: [w444] -> w432
                      n184 = in-place-dvr #19(w431) -> (w456:refnum<class "TEC editor node.lvclass">, w454:errorcluster)
                      n185 = in-place-dvr #20(w430) -> (w457:refnum<class "TEC editor node.lvclass">, w453:errorcluster)
                      n186 = in-place-dvr #21(w429) -> (w450:refnum<class "Engine Parent Editor Node.lvclass">, w449:errorcluster)
                      n187 = in-place-dvr #22(w425) -> (w440:refnum<class "Engine Parent Editor Node.lvclass">, w439:errorcluster)
                      n188 = call <vilib>:"read engine configuration.vi"("error in"=w439, "Engine Parent Editor Node in"=w440) -> ("error out"=w438:errorcluster, "engine configuration"=w434:refnum<class "engine configuration.lvclass">, "Engine Parent Editor Node out"=w441:refnum<class "Engine Parent Editor Node.lvclass">)  [unwired: 7 in]
                      n189 = call <vilib>:"read engine configuration.vi"("error in"=w449, "Engine Parent Editor Node in"=w450) -> ("error out"=w442:errorcluster, "engine configuration"=w446:refnum<class "engine configuration.lvclass">, "Engine Parent Editor Node out"=w448:refnum<class "Engine Parent Editor Node.lvclass">)  [unwired: 7 in]
                      n190 = Merge Errors(w459, w454, w453, w442, w438) -> (w455:errorcluster)
                      n191 = call "unpair modules.vi"("paired engine in"=w434, "error in"=w455, "engine configuration in"=w446, "module to unpair"=w457, "UDP Broadcast Editor Node in"=w456) -> ("error out"=w458:errorcluster, "engine configuration out"=w445:refnum<class "engine configuration.lvclass">, "unpaired module"=w451:refnum<class "TEC editor node.lvclass">, "UDP Broadcast Editor Node out"=w452:refnum<class "TEC editor node.lvclass">, "paired engine out"=w435:refnum<class "engine configuration.lvclass">)  [unwired: 2 in]
                      n192 = call <vilib>:"write engine configuration.vi"("error in"=w438, "engine configuration"=w435, "Engine Parent Editor Node in"=w441) -> ("error out"=w437:errorcluster, "Engine Parent Editor Node out"=w436:refnum<class "Engine Parent Editor Node.lvclass">)  [unwired: 7 in]
                      n193 = call <vilib>:"write engine configuration.vi"("error in"=w442, "engine configuration"=w445, "Engine Parent Editor Node in"=w448) -> ("error out"=w443:errorcluster, "Engine Parent Editor Node out"=w447:refnum<class "Engine Parent Editor Node.lvclass">)  [unwired: 7 in]
                      n194 = Merge Errors(w458, w443, w437) -> (w444:errorcluster)
                      n195 = in-place-dvr #19(w452) -> (w428:errorcluster)  [unwired: 1 out]
                      n196 = in-place-dvr #20(w451) -> (w427:errorcluster)  [unwired: 1 out]
                      n197 = in-place-dvr #21(w447) -> (w426:errorcluster)  [unwired: 1 out]
                      n198 = in-place-dvr #22(w436) -> ()  [unwired: 2 out]
                    }
                    n199 = flat-sequence {
                      tunnel: w428 -> [_]
                      tunnel: w427 -> [_]
                      tunnel: w426 -> [_]
                      frame #0 {
                      }
                    }
                  }
                  frame Error {
                  }
                }
              }
              frame "" {
                # "do nothing if nothing was selected"
              }
            }
          }
        }
        n200 = case shown="Error" w53 {
          selector: w53 -> [w56 w60]
          tunnel: [w57 w61] -> w52
          tunnel: w51 -> [w57 w61]
          tunnel: [w56 w58] -> w50
          frame No Error {
          }
          frame Error {
            n201 = call <vilib>:"Simple Error Handler.vi"("error in (no error)"=w60) -> ("error out"=w59:errorcluster)  [unwired: 4 in, 4 out]
            n202 = call <vilib>:"Clear Errors.vi"("error in (no error)"=w59) -> ("error out"=w58:errorcluster)  [unwired: 6 in]
          }
        }
      }
    }
    frame Error {
    }
  }
  n203 = Unregister For Events(event registration refnum=w29, error in=w28) -> (error out=w24:errorcluster)
  n204 = call <vilib>:"Simple Error Handler.vi"("error in (no error)"=w24) -> ()  [unwired: 4 in, 5 out]
